vi "get image array.vi"(8 "error in (no error)":errorcluster, 11 "Cascade in":refnum<class "Cascade.lvclass">) -> (0 "error out":errorcluster, 3 "Cascade out":refnum<class "Cascade.lvclass">)   [LabVIEW 2012, in "Cascade.lvclass"]
uses:
  Cascade.lvclass
  Cascade.lvclass/Cascade.ctl
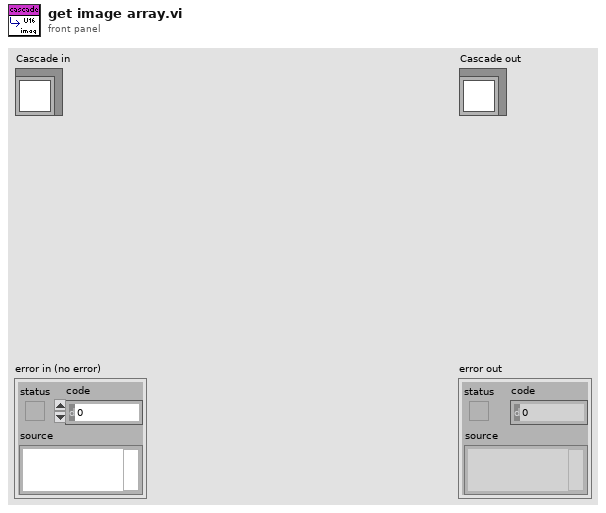
[diagram p1: front panel]
types:
  T1 = typedef "IMAQ Image.ctl" = refnum<image>
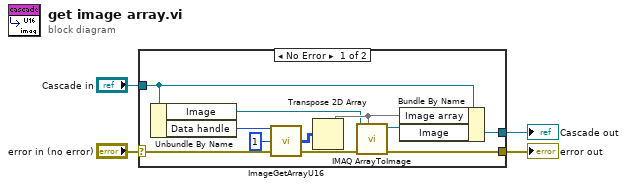
[diagram p0: block diagram]
diagram:
  n1 = case shown="No Error" "error in (no error)" {
    selector: "error in (no error)" -> [w15 w17]
    tunnel: [w9 w17] -> w3
    tunnel: [w11 w16] -> w1
    tunnel: "Cascade in" -> [w12 w16]
    frame No Error {
      n2 = Unbundle By Name(w12) -> ("Image"=w6:T1, "Data handle"=w14:u32)
      n3 = call <userlib>:"ImageGetArrayU16.vi"("error in"=w15, "Z position"=u32 1, "Image Handle"=w14) -> ("error out"=w10:errorcluster, "Array uint 16"=w8:u16[][])  [unwired: 1 out]
      n4 = Transpose 2D Array(2D array=w8) -> (transposed array=w7:u16[][])
      n5 = call "IMAQ ArrayToImage"("Image Pixels (U16)"=w7, "error in (no error)"=w10, "Image"=w6) -> ("error out"=w9:errorcluster, "Image Out"=w5:T1)  [unwired: 7 in]
      n6 = Bundle By Name(cluster=w12, "Image array"=w7, "Image"=w5) -> (w11:refnum<class "Cascade.lvclass">)
    }
    frame Error {
    }
  }
  "error out" <- w3
  "Cascade out" <- w1
